vi "SetAmPhase.vi"(4 "b_am":fxp<+/-,16,2>, 6 "a_am":fxp<+/-,16,2>, 8 "error in (no error)":errorcluster, 9 "fclk (MHz)":dbl=10.0 format="%#_13g", 10 "Am freq [kHz]":dbl=10.0, 11 "Scope5785_six_channel":refnum<class "Scope5782_six_channel.lvclass">) -> (0 "error out":errorcluster, 3 "Scope5785_six_channel out":refnum<class "Scope5782_six_channel.lvclass">)   [LabVIEW 2018, in "Scope5782_six_channel.lvclass"]
uses:
  Scope5782_six_channel.lvclass
  FPGA/fpga_settings.ctl
  Scope5782_six_channel.lvclass/Scope5782_six_channel.ctl
  FpgaRef/FpgaRef5782/FpgaRef5782.lvclass
  C:/PXIe/InProgress/source/Host/FpgaRef/FpgaRefBase/FpgaRefBase.lvclass
  <vilib>/rvi/FXPMathLib/FxpInterpret/XNode/nifxpmath_Interpret.xnode
  FpgaRef/FpgaRefBase/FpgaRefBase.lvclass
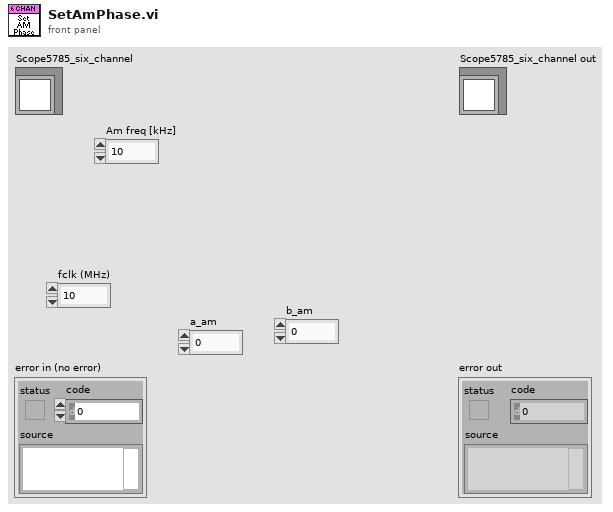
[diagram p1: front panel]
types:
  T1 = typedef "fpga_settings.ctl" = enum16{"Feedback Enable", "New FIR coeffs", "FIR shift", "Enable filter", "Set Downsample", "Downsample", "CIC Gain", "Record length", "Trigger samples", "Quiet time", "a_am", "b_am", "Use fixed delay", "fixed sin_fi", "fixed cos_fi", "Ki*Tau", "Kp", "Kd_Tau", "Fi_start", "Fi_delta", "DC_offs 0", "DC_offs 1", "DC_offs 2", "DC_offs 3", "Ki*Tau am", "Kp am", "Kd_Tau am", "Feedback AM", "Trigger delay", "Feedback delay", "Setpoint enable", "Beam enable", "Samples to acquire", "Cavity Enable", "Cavity C1", "Cavity C2", "Cavity C3", "Cavity C4", "Cavity C5", "Input delay", "Ki*Tau Q", "Kp Q", "Kd_Tau Q", "Adaptive FF enable", "Feedforward a0", "Feedforward b0", "FF src adress", "FF dest adress", "Output scale", "Input scale", "Host scale", "FF_IIR b0", "FF_IIR b1", "FF_IIR b2", "FF_IIR-a1", "FF_IIR-a2", "Enable HW trigger", "Virtual cavity", "Samples to skip", "Samples to skip 2", "Samples to skip 3", "Cavity C3_2", "Cavity C4_2", "Cavity C5_2", "Cavity C3_3", "Cavity C4_3", "Cavity C5_3", "Cavity_w0_dt", "Piezo setting", "Quench t0", "Quench tau set", "Quench enabled", "Quench reset", "PID enabled I", "PID enabled Q", "Cavity filter a", "Cavity filter b", "Disable e(n)", "FF e(n) src address", "FF first address", "FF last address", "FF PID first address", "FF PID last address", "Quench max output"}
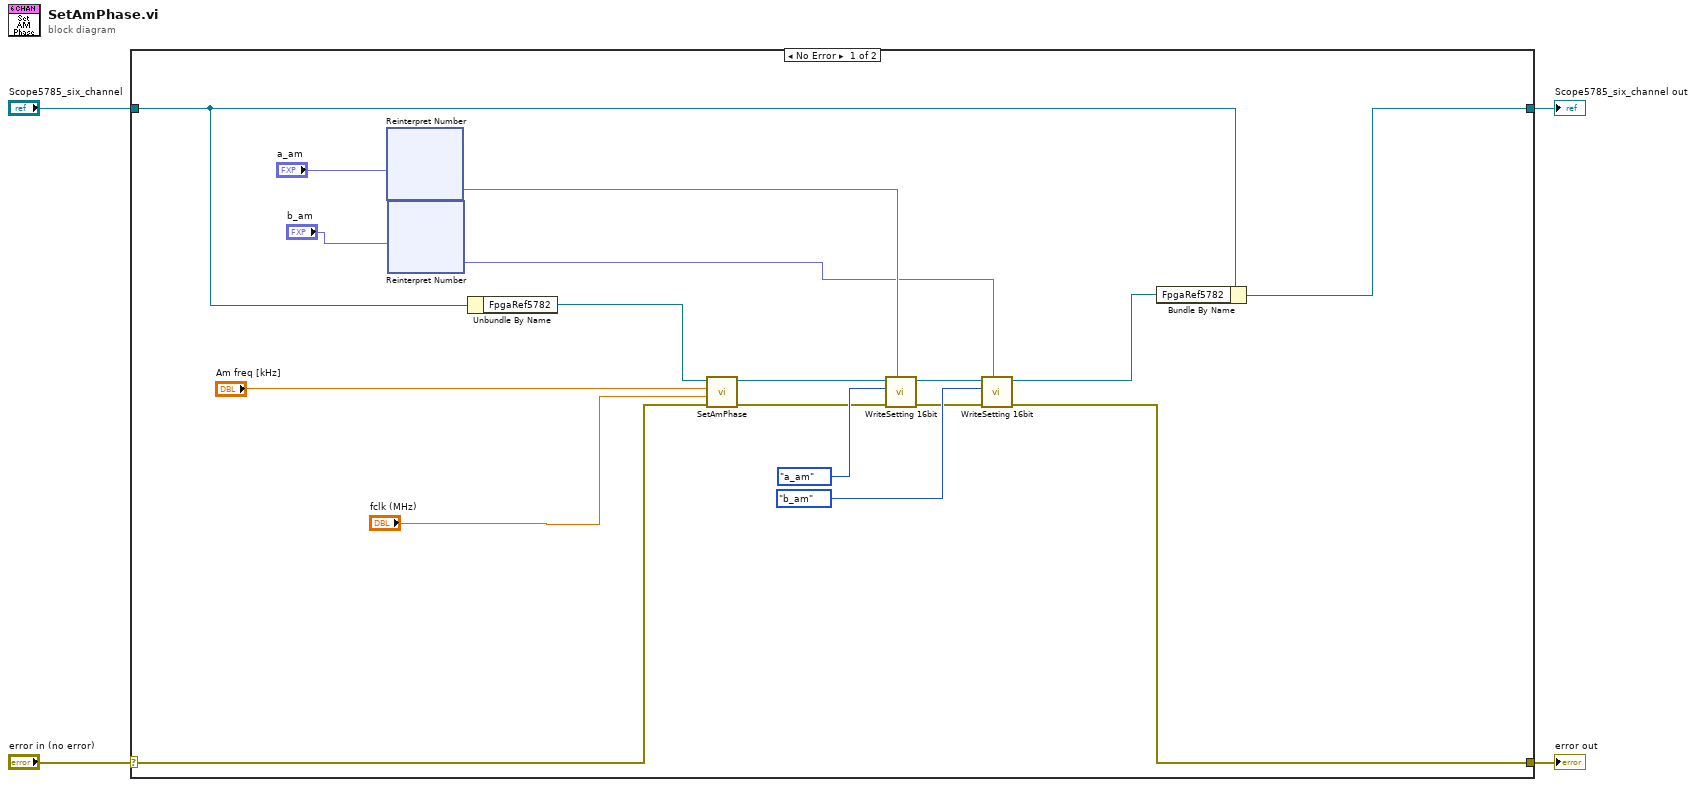
[diagram p0: block diagram]
diagram:
  n1 = case shown="No Error" "error in (no error)" {
    selector: "error in (no error)" -> [w7 w24]
    tunnel: [w6 w24] -> w3
    tunnel: [w11 w23] -> w1
    tunnel: "Scope5785_six_channel" -> [w21 w23]
    frame No Error {
      n2 = xnode "Reinterpret Number"("x"="a_am") -> ("y"=w19:fxp<+,16,16>)
      n3 = xnode "Reinterpret Number"("x"="b_am") -> ("y"=w18:fxp<+,16,16>)
      n4 = Unbundle By Name(w21) -> ("FpgaRef5782"=w15:refnum<class "FpgaRef5782.lvclass">)
      n5 = call "SetAmPhase.vi"("error in (no error)"=w7, "fclk (MHz)"="fclk (MHz)", "Am freq [kHz]"="Am freq [kHz]", "FpgaRef5782 in"=w15) -> ("error out"=w9:errorcluster, "FpgaRef5782 out"=w10:refnum<class "FpgaRef5782.lvclass">)  [unwired: 6 in]
      n6 = call "WriteSetting 16bit.vi"("value"=w19, "error in (no error)"=w9, "FPGA Setting"=fpga_settings."a_am", "FpgaRefBase in"=w10) -> ("error out"=w8:errorcluster, "FpgaRefBase out"=w16:refnum<class "FpgaRef5782.lvclass">)  [unwired: 6 in]
      n7 = call "WriteSetting 16bit.vi"("value"=w18, "error in (no error)"=w8, "FPGA Setting"=fpga_settings."b_am", "FpgaRefBase in"=w16) -> ("error out"=w6:errorcluster, "FpgaRefBase out"=w12:refnum<class "FpgaRef5782.lvclass">)  [unwired: 6 in]
      n8 = Bundle By Name(cluster=w21, "FpgaRef5782"=w12) -> (w11:refnum<class "Scope5782_six_channel.lvclass">)
    }
    frame Error {
    }
  }
  "error out" <- w3
  "Scope5785_six_channel out" <- w1
